vi "RPC Method GreeterService GetFeature.vi"(3 "error in (no error)":errorcluster, 4 "gRPCid in":T1, 5 "DNL_LabVIEW Object in":refnum<class "GreeterServiceImpl.lvclass">) -> (0 "error out":errorcluster, 1 "gRPCid out":T1, 2 "DNL_LabVIEW Object out":refnum<class "GreeterServiceImpl.lvclass">)   [LabVIEW 2019, in "UserCode_impl_server.lvlib" / "GreeterServiceImpl.lvclass"]
uses:
  GreeterServiceImpl.lvclass
  <vilib>/gRPC/LabVIEW gRPC Library/Shared/grpcId.ctl
  Generated_stub_server/RPC Messages/Greeter_res.ctl
  Generated_stub_server/RPC Messages/Greeter_res_res_oneof/Greeter_res_res_oneof.lvclass
  Generated_stub_server/RPC Messages/Greeter_req_req_oneof/Greeter_req_req_oneof.lvclass/Greeter_req_req_oneof.ctl
  Generated_stub_server/RPC Messages/Greeter_res_res_oneof/Greeter_res_res_oneof.lvclass/Greeter_res_res_oneof.ctl
  Generated_stub_server/Generated_stub_server.lvlib
  Generated_stub_server/RPC Service/GreeterServiceStub/GreeterServiceStub.lvclass
  Generated_stub_server/RPC Messages/Greeter_req_req_oneof/Greeter_req_req_oneof.lvclass
  <vilib>/gRPC/LabVIEW gRPC Library/grpc-lvsupport-release.lvlib
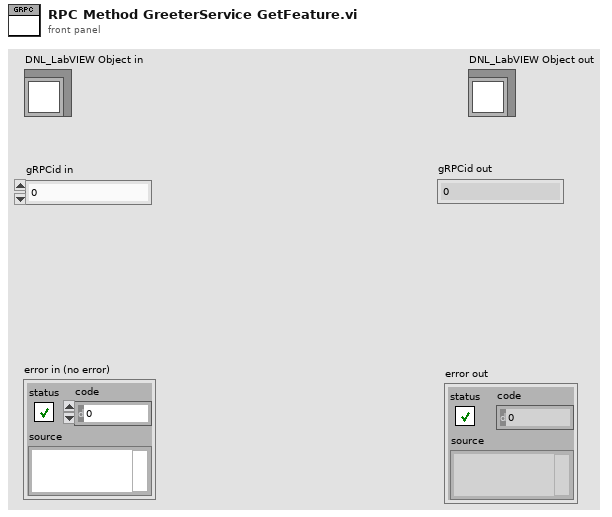
[diagram p1: front panel]
types:
  T1 = typedef "grpc-lvsupport-release.lvlib/grpcId.ctl" = u64
  T2 = typedef "Generated_stub_server.lvlib/Greeter_res.ctl" = cluster{"res_latitude":i32, "Greeter_res_res_oneof":refnum<class "Greeter_res_res_oneof.lvclass">}
  T3 = typedef "Generated_stub_server.lvlib/Greeter_req.ctl" = cluster{"req_latitude":i32, "Greeter_req_req_oneof":refnum<class "Greeter_req_req_oneof.lvclass">}
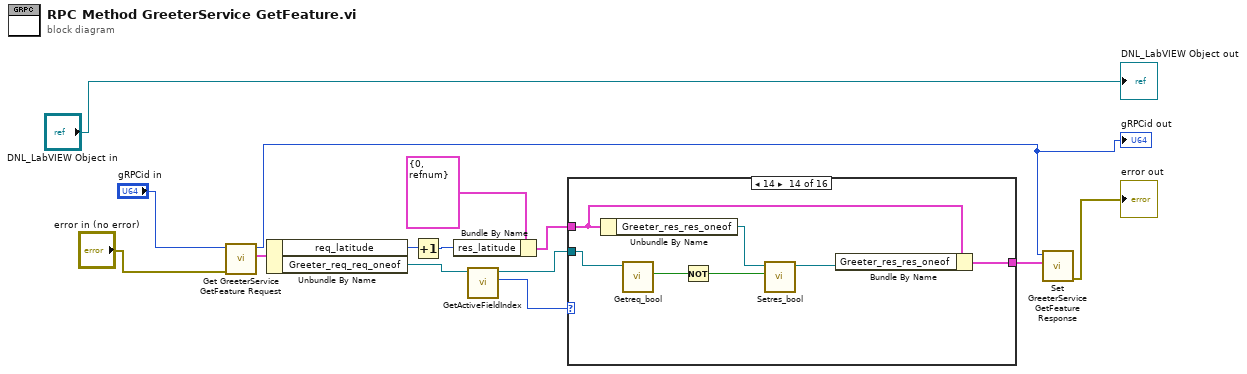
[diagram p0: block diagram]
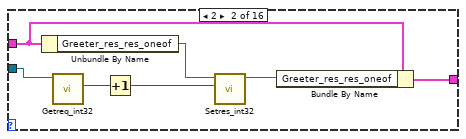
[diagram p3: hidden frame]
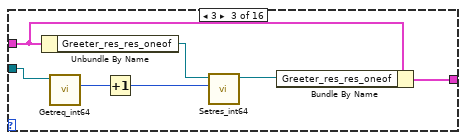
[diagram p4: hidden frame]
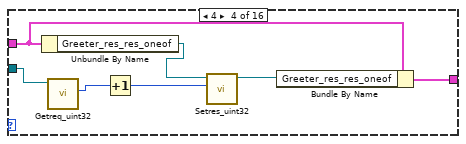
[diagram p5: hidden frame]
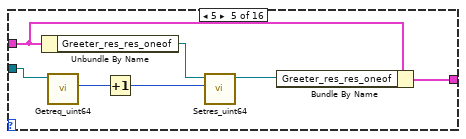
[diagram p6: hidden frame]
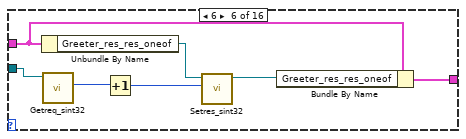
[diagram p7: hidden frame]
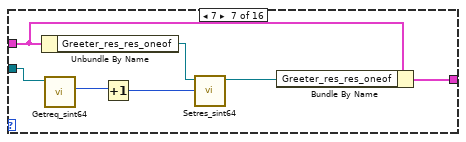
[diagram p8: hidden frame]
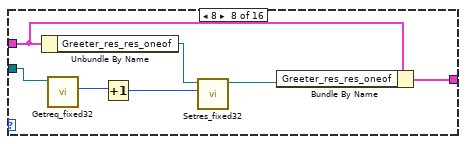
[diagram p9: hidden frame]
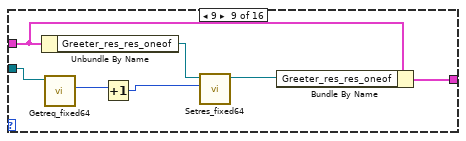
[diagram p10: hidden frame]
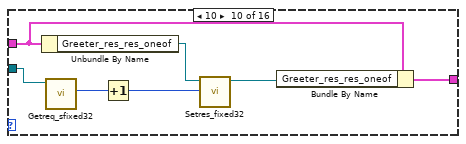
[diagram p11: hidden frame]
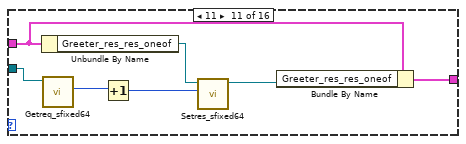
[diagram p12: hidden frame]
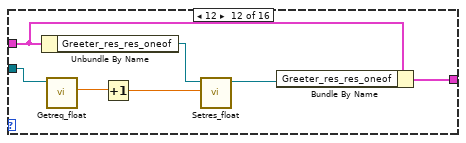
[diagram p13: hidden frame]
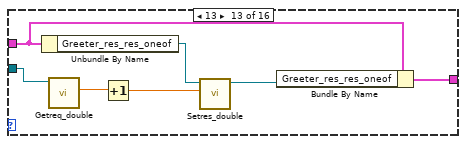
[diagram p14: hidden frame]
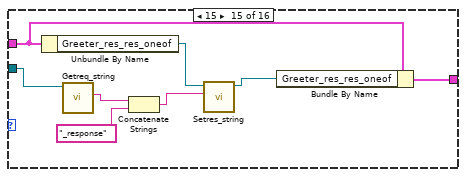
[diagram p15: hidden frame]
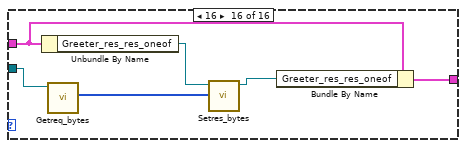
[diagram p16: hidden frame]
diagram:
  n1 = call "Get GreeterService GetFeature Request.vi"("error in (no error)"="error in (no error)", "gRPCid"="gRPCid in") -> ("Message Data"=w14:T3, "gRPCid out"=w2:T1)  [unwired: 7 in, 1 out]
  "gRPCid out" <- w2
  n2 = Unbundle By Name(w14) -> ("req_latitude"=w11:i32, "Greeter_req_req_oneof"=w10:refnum<class "Greeter_req_req_oneof.lvclass">)
  n3 = Increment(x=w11) -> (x+1=w12:i32)
  n4 = Bundle By Name(cluster=T2 {"res_latitude"=0, "Greeter_res_res_oneof"=refnum} ("Greeter_res"), "res_latitude"=w12) -> (w8:T2)
  n5 = call "GetActiveFieldIndex.vi"("OneOfTemplate in"=w10) -> ("Active Field Index"=w9:i32, "OneOfTemplate out"=w7:refnum<class "Greeter_req_req_oneof.lvclass">)  [unwired: 8 in, 1 out]
  n6 = case shown="14" w9 {
    tunnel: w8 -> [w15 w18 w29 w36 w43 w50 w57 w64 w71 w78 w85 w92 w99 w106 w114 w120]
    tunnel: w7 -> [_ w22 w27 w34 w41 w48 w55 w62 w69 w76 w81 w90 w97 w104 w112 w118]
    tunnel: [w15 w16 w28 w35 w42 w49 w56 w63 w70 w77 w84 w91 w98 w105 w113 w119] -> w6
    frame 0, Default {
    }
    frame 2 {
      n7 = Unbundle By Name(w18) -> ("Greeter_res_res_oneof"=w19:refnum<class "Greeter_res_res_oneof.lvclass">)
      n8 = call "Getreq_int32.vi"("OneOfTemplate in"=w22) -> ("Get_Val"=w21:i32)  [unwired: 8 in, 2 out]
      n9 = Increment(x=w21) -> (x+1=w20:i32)
      n10 = call "Setres_int32.vi"("Set_Val"=w20, "OneOfTemplate in"=w19) -> ("OneOfTemplate out"=w17:refnum<class "Greeter_res_res_oneof.lvclass">)  [unwired: 8 in, 1 out]
      n11 = Bundle By Name(cluster=w18, "Greeter_res_res_oneof"=w17) -> (w16:T2)
    }
    frame 3 {
      n12 = Unbundle By Name(w29) -> ("Greeter_res_res_oneof"=w25:refnum<class "Greeter_res_res_oneof.lvclass">)
      n13 = call "Getreq_int64.vi"("OneOfTemplate in"=w27) -> ("Get_Val"=w26:i64)  [unwired: 8 in, 2 out]
      n14 = Increment(x=w26) -> (x+1=w24:i64)
      n15 = call "Setres_int64.vi"("Set_Val"=w24, "OneOfTemplate in"=w25) -> ("OneOfTemplate out"=w23:refnum<class "Greeter_res_res_oneof.lvclass">)  [unwired: 8 in, 1 out]
      n16 = Bundle By Name(cluster=w29, "Greeter_res_res_oneof"=w23) -> (w28:T2)
    }
    frame 4 {
      n17 = Unbundle By Name(w36) -> ("Greeter_res_res_oneof"=w31:refnum<class "Greeter_res_res_oneof.lvclass">)
      n18 = call "Getreq_uint32.vi"("OneOfTemplate in"=w34) -> ("Get_Val"=w33:u32)  [unwired: 8 in, 2 out]
      n19 = Increment(x=w33) -> (x+1=w32:u32)
      n20 = call "Setres_uint32.vi"("Set_Val"=w32, "OneOfTemplate in"=w31) -> ("OneOfTemplate out"=w30:refnum<class "Greeter_res_res_oneof.lvclass">)  [unwired: 8 in, 1 out]
      n21 = Bundle By Name(cluster=w36, "Greeter_res_res_oneof"=w30) -> (w35:T2)
    }
    frame 5 {
      n22 = Unbundle By Name(w43) -> ("Greeter_res_res_oneof"=w38:refnum<class "Greeter_res_res_oneof.lvclass">)
      n23 = call "Getreq_uint64.vi"("OneOfTemplate in"=w41) -> ("Get_Val"=w40:u64)  [unwired: 8 in, 2 out]
      n24 = Increment(x=w40) -> (x+1=w39:u64)
      n25 = call "Setres_uint64.vi"("Set_Val"=w39, "OneOfTemplate in"=w38) -> ("OneOfTemplate out"=w37:refnum<class "Greeter_res_res_oneof.lvclass">)  [unwired: 8 in, 1 out]
      n26 = Bundle By Name(cluster=w43, "Greeter_res_res_oneof"=w37) -> (w42:T2)
    }
    frame 6 {
      n27 = Unbundle By Name(w50) -> ("Greeter_res_res_oneof"=w45:refnum<class "Greeter_res_res_oneof.lvclass">)
      n28 = call "Getreq_sint32.vi"("OneOfTemplate in"=w48) -> ("Get_Val"=w47:i32)  [unwired: 8 in, 2 out]
      n29 = Increment(x=w47) -> (x+1=w46:i32)
      n30 = call "Setres_sint32.vi"("Set_Val"=w46, "OneOfTemplate in"=w45) -> ("OneOfTemplate out"=w44:refnum<class "Greeter_res_res_oneof.lvclass">)  [unwired: 8 in, 1 out]
      n31 = Bundle By Name(cluster=w50, "Greeter_res_res_oneof"=w44) -> (w49:T2)
    }
    frame 7 {
      n32 = Unbundle By Name(w57) -> ("Greeter_res_res_oneof"=w52:refnum<class "Greeter_res_res_oneof.lvclass">)
      n33 = call "Getreq_sint64.vi"("OneOfTemplate in"=w55) -> ("Get_Val"=w54:i64)  [unwired: 8 in, 2 out]
      n34 = Increment(x=w54) -> (x+1=w53:i64)
      n35 = call "Setres_sint64.vi"("Set_Val"=w53, "OneOfTemplate in"=w52) -> ("OneOfTemplate out"=w51:refnum<class "Greeter_res_res_oneof.lvclass">)  [unwired: 8 in, 1 out]
      n36 = Bundle By Name(cluster=w57, "Greeter_res_res_oneof"=w51) -> (w56:T2)
    }
    frame 8 {
      n37 = Unbundle By Name(w64) -> ("Greeter_res_res_oneof"=w59:refnum<class "Greeter_res_res_oneof.lvclass">)
      n38 = call "Getreq_fixed32.vi"("OneOfTemplate in"=w62) -> ("Get_Val"=w61:u32)  [unwired: 8 in, 2 out]
      n39 = Increment(x=w61) -> (x+1=w60:u32)
      n40 = call "Setres_fixed32.vi"("Set_Val"=w60, "OneOfTemplate in"=w59) -> ("OneOfTemplate out"=w58:refnum<class "Greeter_res_res_oneof.lvclass">)  [unwired: 8 in, 1 out]
      n41 = Bundle By Name(cluster=w64, "Greeter_res_res_oneof"=w58) -> (w63:T2)
    }
    frame 9 {
      n42 = Unbundle By Name(w71) -> ("Greeter_res_res_oneof"=w66:refnum<class "Greeter_res_res_oneof.lvclass">)
      n43 = call "Getreq_fixed64.vi"("OneOfTemplate in"=w69) -> ("Get_Val"=w68:u64)  [unwired: 8 in, 2 out]
      n44 = Increment(x=w68) -> (x+1=w67:u64)
      n45 = call "Setres_fixed64.vi"("Set_Val"=w67, "OneOfTemplate in"=w66) -> ("OneOfTemplate out"=w65:refnum<class "Greeter_res_res_oneof.lvclass">)  [unwired: 8 in, 1 out]
      n46 = Bundle By Name(cluster=w71, "Greeter_res_res_oneof"=w65) -> (w70:T2)
    }
    frame 10 {
      n47 = Unbundle By Name(w78) -> ("Greeter_res_res_oneof"=w73:refnum<class "Greeter_res_res_oneof.lvclass">)
      n48 = call "Getreq_sfixed32.vi"("OneOfTemplate in"=w76) -> ("Get_Val"=w75:i32)  [unwired: 8 in, 2 out]
      n49 = Increment(x=w75) -> (x+1=w74:i32)
      n50 = call "Setres_fixed32.vi"("Set_Val"=w74, "OneOfTemplate in"=w73) -> ("OneOfTemplate out"=w72:refnum<class "Greeter_res_res_oneof.lvclass">)  [unwired: 8 in, 1 out]
      n51 = Bundle By Name(cluster=w78, "Greeter_res_res_oneof"=w72) -> (w77:T2)
    }
    frame 11 {
      n52 = Unbundle By Name(w85) -> ("Greeter_res_res_oneof"=w80:refnum<class "Greeter_res_res_oneof.lvclass">)
      n53 = call "Getreq_sfixed64.vi"("OneOfTemplate in"=w81) -> ("Get_Val"=w83:i64)  [unwired: 8 in, 2 out]
      n54 = Increment(x=w83) -> (x+1=w82:i64)
      n55 = call "Setres_sfixed64.vi"("Set_Val"=w82, "OneOfTemplate in"=w80) -> ("OneOfTemplate out"=w79:refnum<class "Greeter_res_res_oneof.lvclass">)  [unwired: 8 in, 1 out]
      n56 = Bundle By Name(cluster=w85, "Greeter_res_res_oneof"=w79) -> (w84:T2)
    }
    frame 12 {
      n57 = Unbundle By Name(w92) -> ("Greeter_res_res_oneof"=w87:refnum<class "Greeter_res_res_oneof.lvclass">)
      n58 = call "Getreq_float.vi"("OneOfTemplate in"=w90) -> ("Get_Val"=w89:sgl)  [unwired: 8 in, 2 out]
      n59 = Increment(x=w89) -> (x+1=w88:sgl)
      n60 = call "Setres_float.vi"("Set_Val"=w88, "OneOfTemplate in"=w87) -> ("OneOfTemplate out"=w86:refnum<class "Greeter_res_res_oneof.lvclass">)  [unwired: 8 in, 1 out]
      n61 = Bundle By Name(cluster=w92, "Greeter_res_res_oneof"=w86) -> (w91:T2)
    }
    frame 13 {
      n62 = Unbundle By Name(w99) -> ("Greeter_res_res_oneof"=w94:refnum<class "Greeter_res_res_oneof.lvclass">)
      n63 = call "Getreq_double.vi"("OneOfTemplate in"=w97) -> ("Get_Val"=w96:dbl)  [unwired: 8 in, 2 out]
      n64 = Increment(x=w96) -> (x+1=w95:dbl)
      n65 = call "Setres_double.vi"("Set_Val"=w95, "OneOfTemplate in"=w94) -> ("OneOfTemplate out"=w93:refnum<class "Greeter_res_res_oneof.lvclass">)  [unwired: 8 in, 1 out]
      n66 = Bundle By Name(cluster=w99, "Greeter_res_res_oneof"=w93) -> (w98:T2)
    }
    frame 14 {
      n67 = Unbundle By Name(w106) -> ("Greeter_res_res_oneof"=w101:refnum<class "Greeter_res_res_oneof.lvclass">)
      n68 = call "Getreq_bool.vi"("OneOfTemplate in"=w104) -> ("Get_Val"=w103:bool)  [unwired: 8 in, 2 out]
      n69 = Not(x=w103) -> (.not. x?=w102:bool)
      n70 = call "Setres_bool.vi"("Set_Val"=w102, "OneOfTemplate in"=w101) -> ("OneOfTemplate out"=w100:refnum<class "Greeter_res_res_oneof.lvclass">)  [unwired: 8 in, 1 out]
      n71 = Bundle By Name(cluster=w106, "Greeter_res_res_oneof"=w100) -> (w105:T2)
    }
    frame 15 {
      n72 = Unbundle By Name(w114) -> ("Greeter_res_res_oneof"=w108:refnum<class "Greeter_res_res_oneof.lvclass">)
      n73 = call "Getreq_string.vi"("OneOfTemplate in"=w112) -> ("Get_Val"=w110:string)  [unwired: 8 in, 2 out]
      n74 = Concatenate Strings(w110, "_response" ("string")) -> (w109:string)
      n75 = call "Setres_string.vi"("Set_Val"=w109, "OneOfTemplate in"=w108) -> ("OneOfTemplate out"=w107:refnum<class "Greeter_res_res_oneof.lvclass">)  [unwired: 8 in, 1 out]
      n76 = Bundle By Name(cluster=w114, "Greeter_res_res_oneof"=w107) -> (w113:T2)
    }
    frame 16 {
      n77 = Unbundle By Name(w120) -> ("Greeter_res_res_oneof"=w116:refnum<class "Greeter_res_res_oneof.lvclass">)
      n78 = call "Getreq_bytes.vi"("OneOfTemplate in"=w118) -> ("Get_Val"=w117:u8[])  [unwired: 8 in, 2 out]
      n79 = call "Setres_bytes.vi"("Set_Val"=w117, "OneOfTemplate in"=w116) -> ("OneOfTemplate out"=w115:refnum<class "Greeter_res_res_oneof.lvclass">)  [unwired: 8 in, 1 out]
      n80 = Bundle By Name(cluster=w120, "Greeter_res_res_oneof"=w115) -> (w119:T2)
    }
  }
  n81 = call "Set GreeterService GetFeature Response.vi"("Message Data"=w6, "gRPCid in"=w2) -> ("error out"=→"error out":errorcluster)  [unwired: 9 in]
  "DNL_LabVIEW Object out" <- "DNL_LabVIEW Object in"
